vi "Send Response Message.vi"(8 "error in (no error)":errorcluster, 10 "Message":refnum<class "Message.lvclass">, 11 "Actor in":refnum<class "Actor.lvclass">) -> (0 "error out":errorcluster)   [LabVIEW 2015, in "Actor.lvclass"]
uses:
  Actor.lvclass
  Messaging/Message/Message.lvclass
  Actor.lvclass/Actor.ctl
  Messaging/Messenger/Messenger.lvclass/Messenger.ctl
  Messaging/Message/Message.lvclass/Message.ctl
  Messaging/Message/get Priority.vi
  Messaging/Messenger/Messenger.lvclass
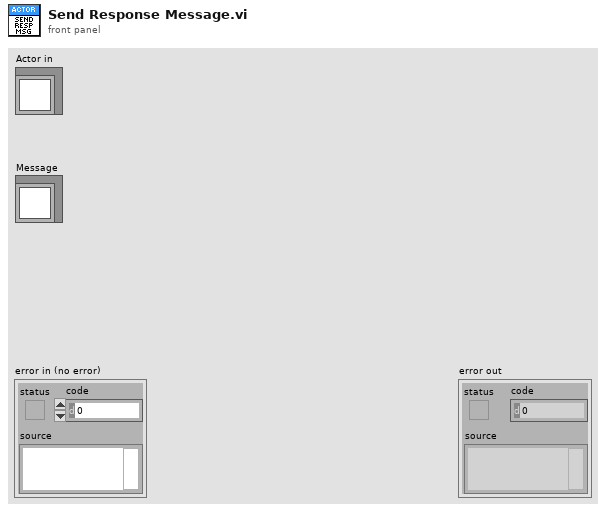
[diagram p1: front panel]
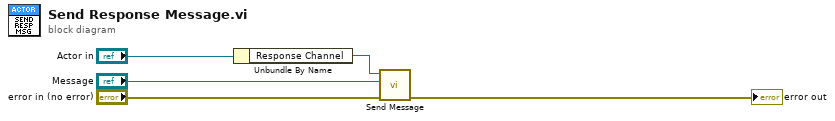
[diagram p0: block diagram]
diagram:
  n1 = Unbundle By Name("Actor in") -> ("Response Channel"=w1:refnum<class "Messenger.lvclass">)
  n2 = call "Send Message.vi"("error in (no error)"="error in (no error)", "Message In"="Message", "Messenger in"=w1) -> ("error out"=→"error out":errorcluster)  [unwired: 8 in]
